vi "Unflatten UIP Value.vi"(10 "String Value":string, 11 "CaptionUIP In":refnum<class "CaptionUIP.lvclass">) -> (0 "Error Out":errorcluster, 3 "CaptionUIP Out":refnum<class "CaptionUIP.lvclass">)   [LabVIEW 2020, in "UIM.lvlib" / "CaptionUIP.lvclass"]
uses:
  CaptionUIP.lvclass
  CaptionUIP.lvclass/CaptionUIP.ctl
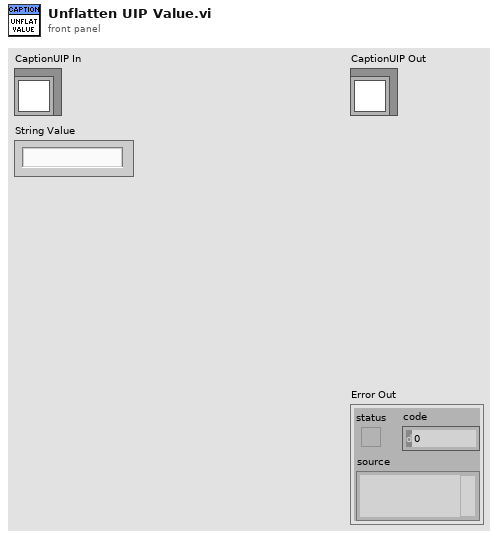
[diagram p1: front panel]
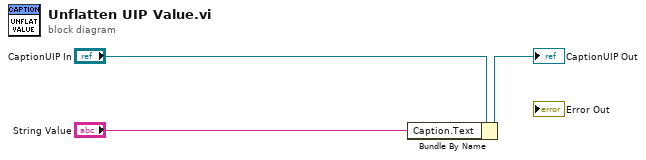
[diagram p0: block diagram]
diagram:
  n1 = Bundle By Name(cluster="CaptionUIP In", "Caption.Text"="String Value") -> (→"CaptionUIP Out":refnum<class "CaptionUIP.lvclass">)
